vi "Fetch Data from 5772 (Raw Data).vi"(7 "Timeout (s)":i32=5, 8 "error in":errorcluster, 10 "Samples":i32=-1, 11 "FPGA VI Reference In":refnum<k20>) -> (0 "error out":errorcluster, 2 "Data Acquired":i16[](array[numeric]), 3 "FPGA VI Reference Out":refnum<k20>, 4 "Elements Remaining":u32)   [LabVIEW 2012]
uses:
  <vilib>/Utility/error.llb/Error Cluster From Error Code.vi
  <vilib>/rvi/errors/niLvFpgaAdjustHostInterfaceError.vi
  <vilib>/rvi/interface/nirviMethod/nirviMethod.xnode
  <vilib>/FPGAPlugInAG/Dynamic/niLvFpga_ReadFifo_Dynamic.vi
  <vilib>/rvi/errors/niLvFpgaMergeErrorWithErrorCode.vi
panel:
  in  "FIFO Type":enum16{"FPGA to Host FIFO (U64)", "Generic"}(ring)
  out "Data":u64[](array[numeric])
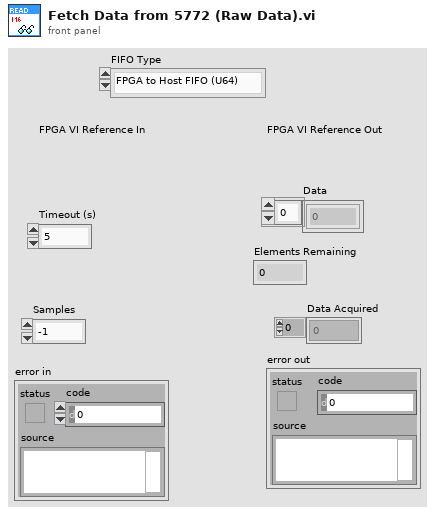
[diagram p1: front panel]
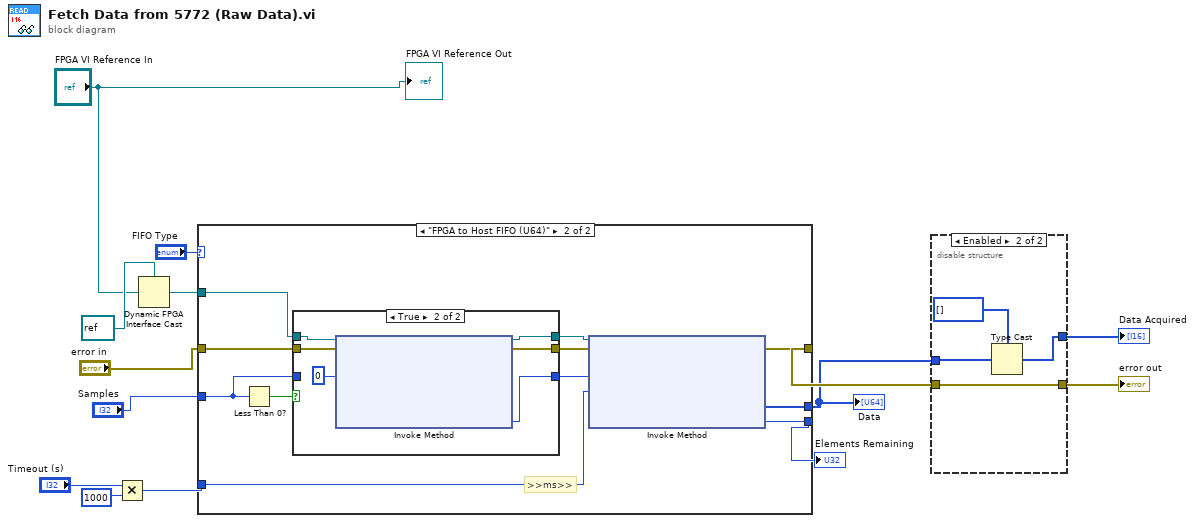
[diagram p0: block diagram]
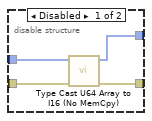
[diagram p2: hidden frame]
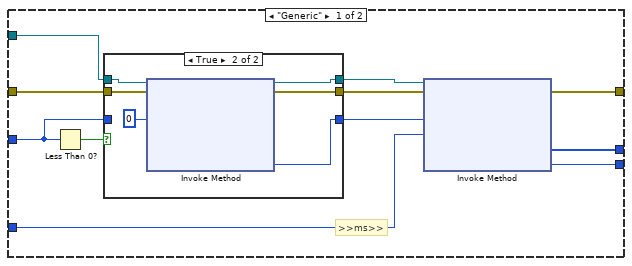
[diagram p3: hidden frame]
diagram:
  n1 = Multiply(x="Timeout (s)", y=1000) -> (x*y=w7:i32)
  n2 = Dynamic FPGA Interface Cast(Session In=refnum<k20> refnum ("Type"), Type="FPGA VI Reference In") -> (Session Out=w11:refnum<k20>)
  n3 = case shown="\"FPGA to Host FIFO (U64)\"" "FIFO Type" {
    tunnel: [w21 w41] -> w3
    tunnel: w11 -> [w20 w40]
    tunnel: [w19 w39] -> w4
    tunnel: [w18 w38] -> w10
    tunnel: "error in" -> [w16 w35]
    tunnel: "Samples" -> [w15 w37]
    tunnel: w7 -> [w17 w36]
    frame "Generic" {
      # ">>ms>>"
      n4 = Less Than 0?(x=w15) -> (x < 0?=w25:bool)
      n5 = case shown="True" w25 {
        tunnel: w20 -> [w28 w34]
        tunnel: w16 -> [w27 w33]
        tunnel: [w28 w32] -> w24
        tunnel: [w27 w31] -> w23
        tunnel: [w26 w30] -> w22
        tunnel: w15 -> [w26 _]
        frame False {
        }
        frame True {
          n6 = xnode "Invoke Method"("FPGA VI Reference In"=w34, "error in"=w33, "Number of Elements"=u32 0) -> ("FPGA VI Reference Out"=w32:refnum<k20>, "error out"=w31:errorcluster, "Elements Remaining"=w30:u32)  [unwired: 1 in, 1 out]
        }
      }
      n7 = xnode "Invoke Method"("FPGA VI Reference In"=w24, "error in"=w23, "Number of Elements"=w22, "Timeout (ms)"=w17) -> ("error out"=w19:errorcluster, "Data"=w21:u64[], "Elements Remaining"=w18:u32)  [unwired: 1 out]
    }
    frame "FPGA to Host FIFO (U64)" {
      # ">>ms>>"
      n8 = Less Than 0?(x=w37) -> (x < 0?=w45:bool)
      n9 = case shown="True" w45 {
        tunnel: w40 -> [w48 w54]
        tunnel: w35 -> [w47 w53]
        tunnel: [w48 w52] -> w44
        tunnel: [w47 w51] -> w43
        tunnel: [w46 w50] -> w42
        tunnel: w37 -> [w46 _]
        frame False {
        }
        frame True {
          n10 = xnode "Invoke Method"("FPGA VI Reference In"=w54, "error in"=w53, "Number of Elements"=u32 0) -> ("FPGA VI Reference Out"=w52:refnum<k20>, "error out"=w51:errorcluster, "Elements Remaining"=w50:u32)  [unwired: 1 in, 1 out]
        }
      }
      n11 = xnode "Invoke Method"("FPGA VI Reference In"=w44, "error in"=w43, "Number of Elements"=w42, "Timeout (ms)"=w36) -> ("error out"=w39:errorcluster, "Data"=w41:u64[], "Elements Remaining"=w38:u32)  [unwired: 1 out]
    }
  }
  "Data" <- w3
  "Elements Remaining" <- w10
  n12 = disable-structure shown="Enabled" {
    disable-tunnel: [w58 w59] -> w14
    disable-tunnel: [w57 w61] -> w13
    disable-tunnel: w4 -> [w56 w59]
    disable-tunnel: w3 -> [w55 w62]
    frame Disabled {
      n13 = call <userlib>:"Type Cast U64 Array to I16 (No MemCpy).vi"("error in"=w56, "Input"=w55) -> ("error out"=w58:errorcluster, "Data Acquired"=w57:i16[])  [unwired: 8 in]
    }
    frame Enabled {
      n14 = Type Cast(type=i16[] [], x=w62) -> (*(type *) &x=w61:i16[])
    }
  }
  "error out" <- w14
  "Data Acquired" <- w13
  "FPGA VI Reference Out" <- "FPGA VI Reference In"
